vi "Display Control Value.vi"(10 "Display Control":T1) -> (2 "DCtrl Value":u8)   [LabVIEW 2020, in "CTI-Visa-DeviceLib.lvlib" / "LCD-I2C.lvclass"]
uses:
  LCD-I2C.lvclass
  LCD-I2C.lvclass/LCD-I2C.ctl
  Display Control.ctl
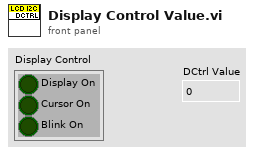
[diagram p1: front panel]
types:
  T1 = typedef "CTI-Visa-DeviceLib.lvlib/LCD-I2C.lvclass/Display Control.ctl" = cluster{"Display On":bool, "Cursor On":bool, "Blink On":bool}
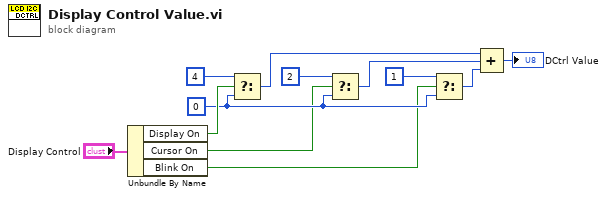
[diagram p0: block diagram]
diagram:
  w7 = u8 0
  n1 = Unbundle By Name("Display Control") -> ("Display On"=w10:bool, "Cursor On"=w6:bool, "Blink On"=w5:bool)
  n2 = Select(t=u8 4, s=w10, f=w7) -> (s? t:f=w4:u8)
  n3 = Select(t=u8 2, s=w6, f=w7) -> (s? t:f=w3:u8)
  n4 = Select(t=u8 1, s=w5, f=w7) -> (s? t:f=w2:u8)
  n5 = Compound Arithmetic op=ADD(w4, w3, w2) -> (→"DCtrl Value":u8)
